vi "Add Value to Database.vi"(8 "error in (no error)":errorcluster, 9 "Array":T1[](array[typedef]), 10 "Measurement Name":string, 11 "Multi Step Database in":refnum<class "Multi Step Database.lvclass">) -> (0 "error out":errorcluster, 3 "Multi Step Database out":refnum<class "Multi Step Database.lvclass">)   [LabVIEW 2016, in "NI Generic Parser.lvlib" / "Multi Step Database.lvclass"]
uses:
  Multi Step Database.lvclass
  Plugins/Measurement Data.lvlibp/Controls/Measurement Description.ctl
  Plugins/String Database.lvlibp/String Database.lvclass
  Plugins/Measurement Data.lvlibp/Controls/Measurement Position.ctl
  Multi Step Database.lvclass/Multi Step Database.ctl
  Private Methods/Read Database.vi
  Private Methods/Write Database.vi
  <vilib>/Utility/error.llb/Error Cluster From Error Code.vi
  <vilib>/ErrorRing/Error Ring.xnode
  Plugins/Measurement Data.lvlibp/Measurement Data.lvclass
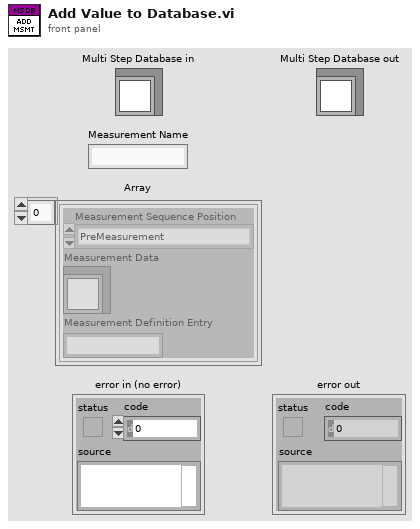
[diagram p1: front panel]
types:
  T1 = typedef "Measurement Data.lvlibp/Measurement Data.lvclass/Measurement Description.ctl" = cluster{"Measurement Sequence Position":T2, "Measurement Data":refnum<class "String Database.lvclass">, "Measurement Definition Entry":string}
  T2 = typedef "Measurement Data.lvlibp/Measurement Data.lvclass/Measurement Position.ctl" = enum16{"PreMeasurement", "MainMeasurement", "PostMeasurement"}
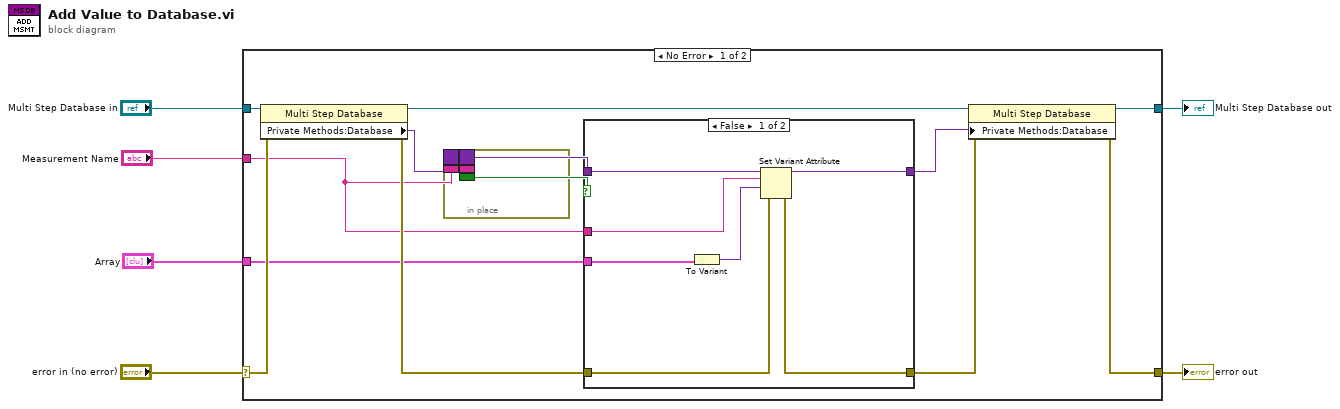
[diagram p0: block diagram]
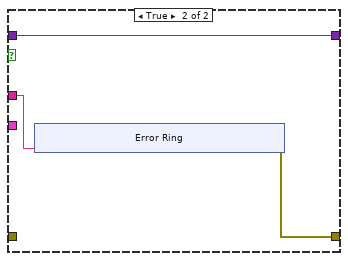
[diagram p2: hidden frame]
diagram:
  n1 = case shown="No Error" "error in (no error)" {
    selector: "error in (no error)" -> [w19 w39]
    tunnel: [w11 w39] -> w5
    tunnel: [w9 w38] -> w3
    tunnel: "Multi Step Database in" -> [w18 w38]
    tunnel: "Measurement Name" -> [w14 _]
    tunnel: "Array" -> [w7 _]
    frame No Error {
      n2 = property class="Multi Step Database"(reference=w18, error in=w19) -> (reference out=w10:refnum<class "Multi Step Database.lvclass">, error out=w16:errorcluster, "Private Methods:Database"=w17:variant)
      n3 = in-place {
        border: w17 -> [_]
        border: w14 -> [_]
        border: [_] -> w12
        border: _ -> [_]
        border: [_] -> w15
      }
      n4 = case shown="False" w15 {
        tunnel: w16 -> [w25 _]
        tunnel: w14 -> [w22 w29]
        tunnel: [w24 w28] -> w13
        tunnel: w12 -> [w26 w27]
        tunnel: [w21 w27] -> w8
        tunnel: w7 -> [w20 _]
        frame False {
          n5 = To Variant(anything=w20) -> (Variant=w23:variant)
          n6 = Set Variant Attribute(Variant=w26, name=w22, value=w23, error in=w25) -> (Variant out=w21:variant, error out=w24:errorcluster)  [unwired: 1 out]
        }
        frame True {
          n7 = xnode "Error Ring"("parameter 0"=w29) -> ("error out"=w28:errorcluster)
        }
      }
      n8 = property class="Multi Step Database"(reference=w10, error in=w13, "Private Methods:Database"=w8) -> (reference out=w9:refnum<class "Multi Step Database.lvclass">, error out=w11:errorcluster)
    }
    frame Error {
    }
  }
  "error out" <- w5
  "Multi Step Database out" <- w3
